vi "Connect.vi"(0 "object in":refnum<class "HPS-17000-PowerModule.lvclass">, 11 "Error In":errorcluster) -> (4 "object out":refnum<class "HPS-17000-PowerModule.lvclass">, 15 "Error Out":errorcluster)   [LabVIEW 2023, in "HPS-17000-PowerModule.lvlib" / "HPS-17000-PowerModule.lvclass"]
uses:
  HPS-17000-PowerModule.lvclass
  <instrlib>/HPS-17000/Client Facing Datatypes/Multi-Cycler Events.ctl
  <instrlib>/HPS-17000/Client Facing Datatypes/Heartbeat Event Data.ctl
  <instrlib>/HPS-17000/Client Facing Datatypes/Faults Event Data.ctl
  <instrlib>/HPS-17000/Client Facing Datatypes/Network Sync Event Data.ctl
  <instrlib>/HPS-17000/Client Facing Datatypes/Setpoint Stream Status Data.ctl
  <instrlib>/HPS-17000/Internal/Find GM ID Single.vi
  <instrlib>/HPS-17000/Internal/Initialize Single.vi
  <instrlib>/HPS-17000/Internal/Initialize Multi.vi
  HPS-17000-PowerModule.lvclass/HPS-17000-PowerModule.ctl
  <instrlib>/HPS-17000/HPS-17000.lvclass
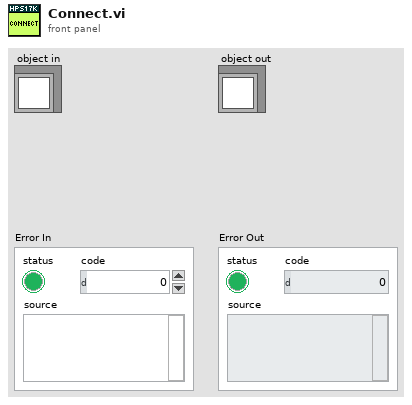
[diagram p1: front panel]
types:
  T1 = typedef "HPS-17000.lvclass/Multi-Cycler Events.ctl" = cluster{"heartbeats events":refnum<user-event>[], "faults events":refnum<user-event>[], "network sync event":refnum<user-event>[], "setpoint status event":refnum<user-event>[]}
  T2 = typedef "HPS-17000-PowerModule.lvlib/HPS-17000-PowerModule.lvclass/ObjectAttributes.ctl" = cluster{"JSON Config Path":path, "Configuration":T3, "GM ID":string, "HPS17000 Refs":refnum<class "HPS-17000.lvclass">[], "connected":bool, "reserved":bool, "events":T1, "nibatterycycler_grpc_Setpoint":T5, "last timestamp":i64, "mode":T6, "range":T7, "measurement array":T8[], "measurement stream":bool, "setpoint stream":bool}
  T3 = typedef "HPS-17000-PowerModule.lvlib/HPS-17000-PowerModule.lvclass/Configuration.ctl" = cluster{"TSN NIC IP Address":string, "HPS17000 IP Addresses":string[], "HPS Topology":enum16{"SINGLE", "MULTI"}, "Setpoint Stream Config":T4, "Measurement Array Size":i32}
  T4 = typedef "Cycler.lvclass/Setpoint Stream Basic Config.ctl" = cluster{"local address":string, "receiver port":u16}
  T5 = typedef "NI_BC_client.lvlib/nibatterycycler_grpc_Setpoint.ctl" = cluster{"voltage":sgl, "current":sgl, "min_power":sgl, "max_power":sgl, "resistance":sgl}
  T6 = typedef "HPS-17000-PowerModule.lvlib/HPS-17000-PowerModule.lvclass/Mode.ctl" = u16
  T7 = typedef "PowerModuleInterface.lvlibp/PowerModuleInterface.lvclass/Range.ctl" = cluster{"Current Max (A)":dbl, "Current Min (A)":dbl, "Voltage Max (V)":dbl, "Voltage Min (V)":dbl}
  T8 = typedef "PowerModuleInterface.lvlibp/PowerModuleInterface.lvclass/Measurements.ctl" = cluster{"measured voltage (V)":dbl, "measured current (A)":dbl, "setpoint voltage (V)":dbl, "setpoint current (A)":dbl, "timestamp":dbl}
  T9 = typedef "HPS-17000.lvclass/Events.ctl" = cluster{"heartbeat failure event":refnum<user-event>, "faults event":refnum<user-event>, "network sync event":refnum<user-event>, "setpoint status event":refnum<user-event>}
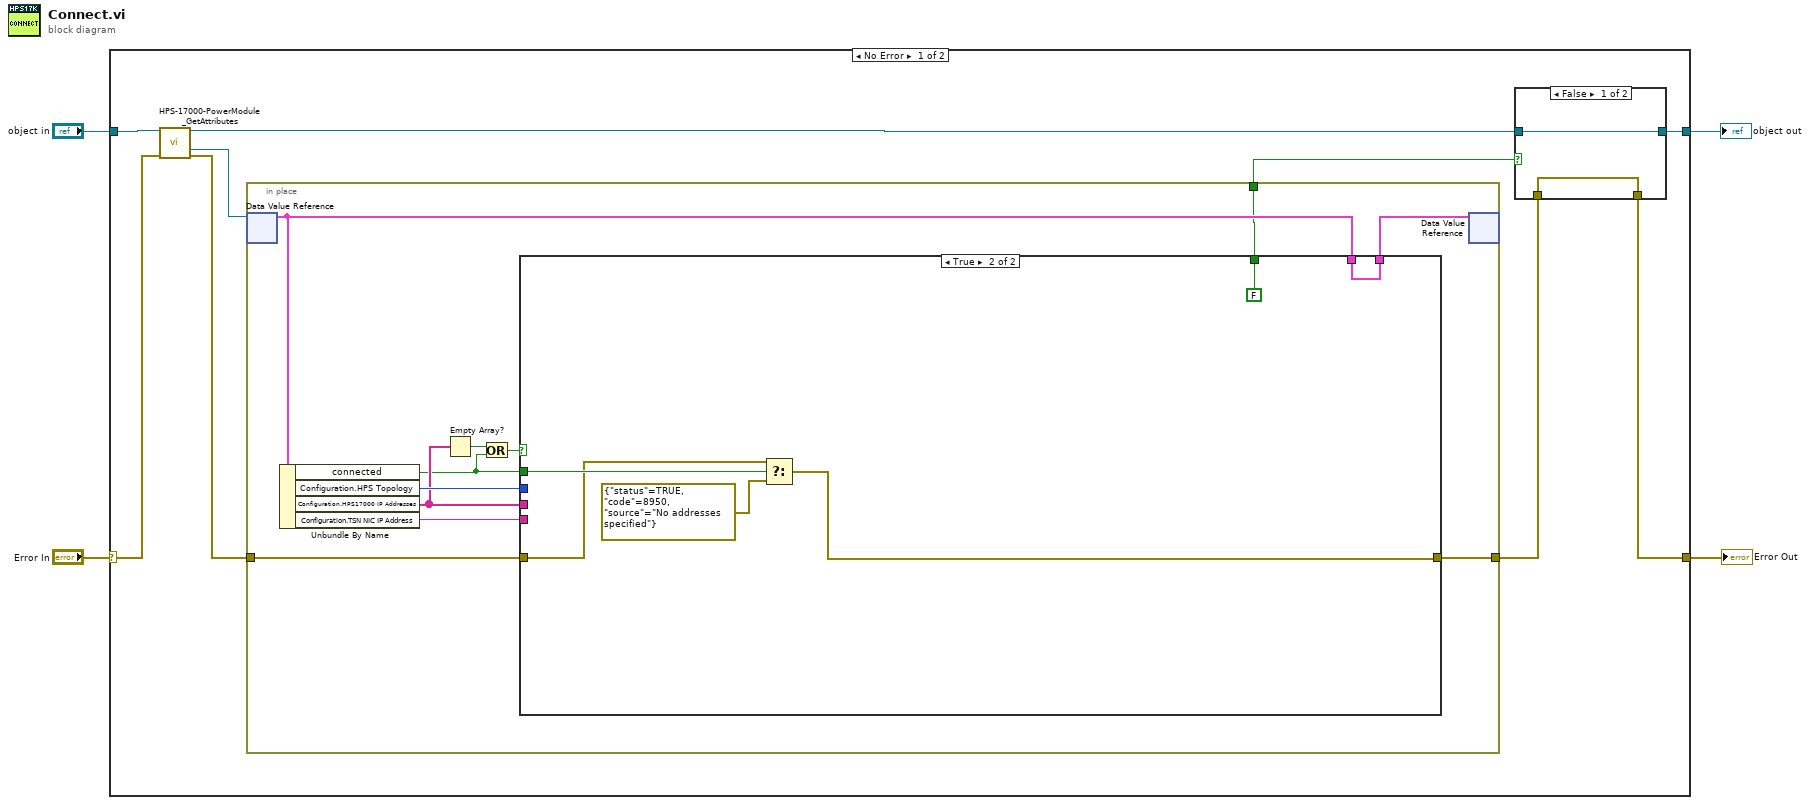
[diagram p0: block diagram]
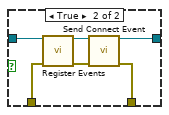
[diagram p2: hidden frame]
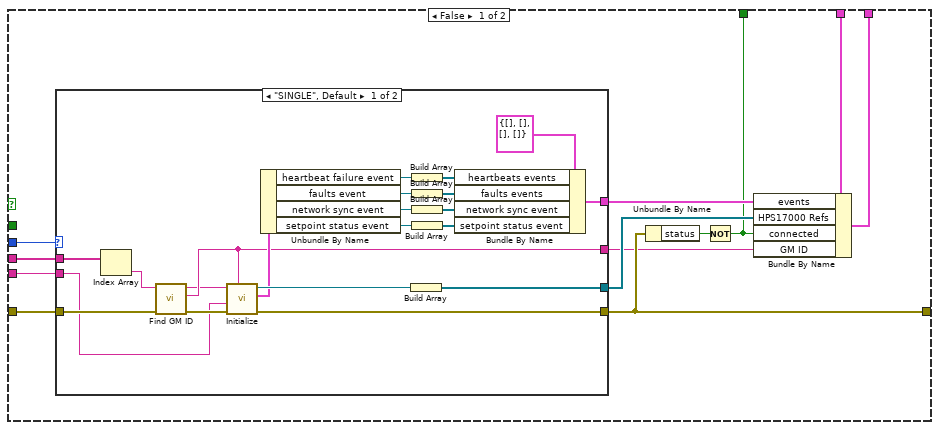
[diagram p3: hidden frame]
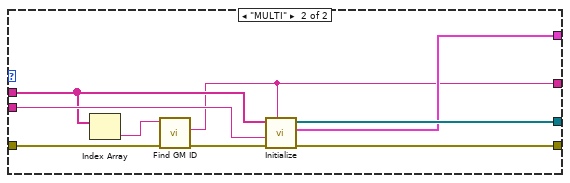
[diagram p4: hidden frame]
diagram:
  n1 = case shown="No Error" "Error In" {
    selector: "Error In" -> [w12 w81]
    tunnel: "object in" -> [w13 w82]
    tunnel: [w6 w82] -> w2
    tunnel: [w7 w81] -> w1
    frame No Error {
      n2 = call "HPS-17000-PowerModule_GetAttributes.vi"("reference in"=w13, "Error In"=w12) -> ("reference out"=w9:refnum<class "HPS-17000-PowerModule.lvclass">, "DataRef"=w11:refnum<data-value>, "Error Out"=w10:errorcluster)  [unwired: 10 in, 1 out]
      n3 = in-place {
        in-place-border: w10 -> [w30]
        in-place-border: [w27] -> w8
        in-place-border: [w26] -> w5
        n4 = in-place-dvr #1(w11) -> (w31:T2)  [unwired: 1 out]
        n5 = Unbundle By Name(w31) -> ("connected"=w22:bool, "Configuration.HPS Topology"=w28:enum16{"SINGLE", "MULTI"}, "Configuration.HPS17000 IP Addresses"=w25:string[], "Configuration.TSN NIC IP Address"=w29:string)
        n6 = Empty Array?(array=w25) -> (empty?=w23:bool)
        n7 = Or(x=w23, y=w22) -> (x .or. y?=w24:bool)
        n8 = case shown="True" w24 {
          tunnel: [w44 w80] -> w32
          tunnel: w31 -> [w43 w80]
          tunnel: w30 -> [w42 w77]
          tunnel: w25 -> [w41 _]
          tunnel: w29 -> [w40 _]
          tunnel: w28 -> [w37 _]
          tunnel: [w36 w76] -> w27
          tunnel: [w33 FALSE] -> w26
          tunnel: w22 -> [_ w78]
          frame False {
            n9 = case shown="\"SINGLE\", Default" w37 {
              tunnel: [w63 w74] -> w38
              tunnel: [w52 w72] -> w39
              tunnel: w41 -> [w51 w69]
              tunnel: w42 -> [w50 w70]
              tunnel: [w65 w73] -> w36
              tunnel: w40 -> [w47 w71]
              tunnel: [w46 w66] -> w34
              frame "SINGLE", Default {
                n10 = Index Array(array=w51) -> (element=w49:string)  [unwired: 1 in]
                n11 = call-poly <instrlib>:"Find GM ID.vi"("error in"=w50, "cycler IP address in"=w49) -> ("error out"=w48:errorcluster, "GM ID"=w46:string, "cycler IP address out"=w45:string)  [unwired: 7 in]
                n12 = call-poly <instrlib>:"Initialize.vi"("intended GM ID"=w46, "error in"=w48, "TSN NIC IP address"=w47, "cycler IP address"=w45) -> ("error out"=w65:errorcluster, "events"=w62:T9, "HPS-17000 out"=w64:refnum<class "HPS-17000.lvclass">)  [unwired: 5 in]
                n13 = Unbundle By Name(w62) -> ("heartbeat failure event"=w60:refnum<user-event>, "faults event"=w58:refnum<user-event>, "network sync event"=w56:refnum<user-event>, "setpoint status event"=w54:refnum<user-event>)
                n14 = Build Array(w64) -> (w63:refnum<class "HPS-17000.lvclass">[])
                n15 = Build Array(w60) -> (w59:refnum<user-event>[])
                n16 = Build Array(w58) -> (w57:refnum<user-event>[])
                n17 = Build Array(w56) -> (w55:refnum<user-event>[])
                n18 = Build Array(w54) -> (w53:refnum<user-event>[])
                n19 = Bundle By Name(cluster=T1 {"heartbeats events"=[], "faults events"=[], "network sync event"=[], "setpoint status event"=[]} ("events"), "heartbeats events"=w59, "faults events"=w57, "network sync event"=w55, "setpoint status event"=w53) -> (w52:T1)
              }
              frame "MULTI" {
                n20 = Index Array(array=w69) -> (element=w68:string)  [unwired: 1 in]
                n21 = call-poly <instrlib>:"Find GM ID.vi"("error in"=w70, "cycler IP address in"=w68) -> ("error out"=w67:errorcluster, "GM ID"=w66:string)  [unwired: 7 in, 1 out]
                n22 = call-poly <instrlib>:"Initialize.vi"("intended GM ID"=w66, "error in"=w67, "TSN NIC IP address"=w71, "cycler IP addresses"=w69) -> ("error out"=w73:errorcluster, "events"=w72:T1, "cycler refs out"=w74:refnum<class "HPS-17000.lvclass">[])  [unwired: 5 in]
              }
            }
            n23 = Unbundle By Name(w36) -> ("status"=w35:bool)
            n24 = Not(x=w35) -> (.not. x?=w33:bool)
            n25 = Bundle By Name(cluster=w43, "events"=w39, "HPS17000 Refs"=w38, "connected"=w33, "GM ID"=w34) -> (w44:T2)
          }
          frame True {
            n26 = Select(t=w77, s=w78, f=errorcluster {"status"=TRUE, "code"=8950, "source"="No addresses specified"}) -> (s? t:f=w76:errorcluster)
          }
        }
        n27 = in-place-dvr #1(w32) -> ()  [unwired: 2 out]
      }
      n28 = case shown="False" w5 {
        tunnel: w9 -> [w14 w21]
        tunnel: w8 -> [w15 w20]
        tunnel: [w15 w17] -> w7
        tunnel: [w14 w16] -> w6
        frame False {
        }
        frame True {
          n29 = call "Register Events.vi"("reference in"=w21, "Error In"=w20) -> ("reference out"=w18:refnum<class "HPS-17000-PowerModule.lvclass">, "Error Out"=w19:errorcluster)  [unwired: 12 in]
          n30 = call "Send Connect Event.vi"("reference in"=w18, "Error In"=w19) -> ("reference out"=w16:refnum<class "HPS-17000-PowerModule.lvclass">, "Error Out"=w17:errorcluster)  [unwired: 12 in]
        }
      }
    }
    frame Error {
    }
  }
  "Error Out" <- w1
  "object out" <- w2
